vi "Make DLL Param(Profile Info).vi"(1 "Profile Info":T1) -> (0 "DLL Parameter":T2)   [LabVIEW 2014, in "Keyence LJ-V7000.lvlib"]
uses:
  Keyence LJ-V7000.lvlib
  Public/Clusters/Profile Info.ctl
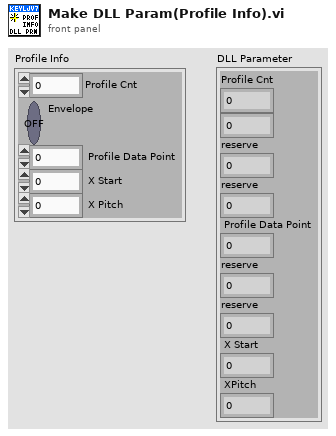
[diagram p1: front panel]
types:
  T1 = typedef "Keyence LJ-V7000.lvlib/Profile Info.ctl" = cluster{"Profile Cnt":u8, "Envelope":bool, " Profile Data Point":u16, " X Start":i32, " X Pitch":i32}
  T2 = cluster{"Profile Cnt":u8, u8, "reserve":u8, "reserve":u8, " Profile Data Point":u16, "reserve":u8, "reserve":u8, " X Start":i32, " XPitch":i32}
  T3 = cluster{"Profile Cnt":u8, u8, "reserve":u8, "reserve":u8, " Profile Data Point":u16, "reserve":u8, "reserve":u8, " X Start":i32, " X Pitch":i32}
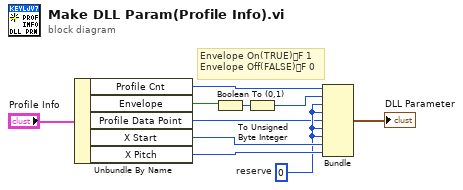
[diagram p0: block diagram]
diagram:
  w7 = u8 0  # reserve
  # "Envelope On(TRUE)F 1\nEnvelope Off(FALSE)F 0"
  n1 = Unbundle By Name("Profile Info") -> ("Profile Cnt"=w2:u8, "Envelope"=w3:bool, "Profile Data Point"=w6:u16, "X Start"=w8:i32, "X Pitch"=w9:i32)
  n2 = Boolean To (0,1)(Boolean=w3) -> (0, 1=w4:i16)
  n3 = To Unsigned Byte Integer(number=w4) -> (unsigned 8bit integer=w5:u8)
  n4 = Bundle("Profile Cnt"=w2, w5, "reserve"=w7, "reserve"=w7, "Profile Data Point"=w6, "reserve"=w7, "reserve"=w7, "X Start"=w8, "X Pitch"=w9) -> (→"DLL Parameter":T3)  [unwired: 1 in]
